vi "Stop Device.vi"(8 "error in":errorcluster, 11 "Configurable Device in":refnum<class "Configurable Device.lvclass">) -> (0 "error out":errorcluster, 3 "Configurable Device out":refnum<class "Configurable Device.lvclass">)   [LabVIEW 2014, in "Device.lvlib" / "Configurable Device.lvclass"]
uses:
  Configurable Device.lvclass
  reusable/Session APIs/File Access/Config Data/Config Data.lvclass
  reusable/Session APIs/Session Log/System Log.lvclass
  Configurable Device.lvclass/Configurable Device.ctl
  <userlib>/_Session Fwk/Session - Root.lvclass
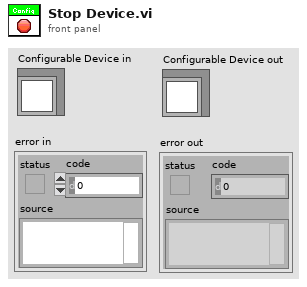
[diagram p1: front panel]
types:
  T1 = typedef "Config Data.lvclass/Config Session.ctl" = refnum<data-value>
  T2 = typedef "Session - Root.lvclass/Session Handle.ctl" = refnum<data-value>
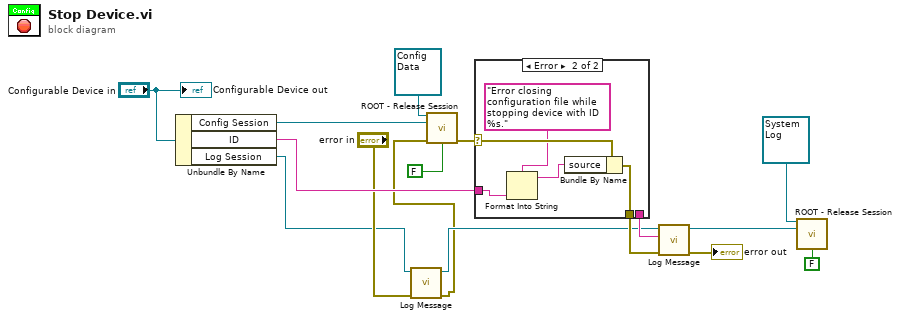
[diagram p0: block diagram]
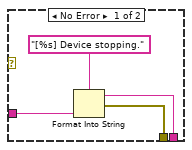
[diagram p2: hidden frame]
diagram:
  n1 = Unbundle By Name("Configurable Device in") -> ("Config Session"=w15:T1, "ID"=w13:string, "Log Session"=w3:T2)
  n2 = call "Log Message.vi"("error in"="error in", "session in"=w3) -> ("error out"=w1:errorcluster, "session out"=w2:T2)  [unwired: 8 in]
  n3 = call <userlib>:"ROOT - Release Session.vi"("OBJ - Session in"=refnum<class "Config Data.lvclass"> refnum ("Config Data"), "Session Handle in"=w15, "error in (no error)"=w1, "force destroy? (F)"=FALSE) -> ("error out"=w6:errorcluster)  [unwired: 10 in, 1 out]
  n4 = case shown="Error" w6 {
    selector: w6 -> [_ w24]
    tunnel: w13 -> [w19 w23]
    tunnel: [w18 w25] -> w12
    tunnel: [w17 _] -> w11
    frame No Error {
      n5 = Format Into String(format string="[%s] Device stopping.", w19) -> (resulting string=w17:string, error out=w18:errorcluster)  [unwired: 2 in]
    }
    frame Error {
      n6 = Format Into String(format string="Error closing configuration file while stopping device with ID %s.", w23) -> (resulting string=w21:string)  [unwired: 2 in, 1 out]
      n7 = Bundle By Name(cluster=w24, "source"=w21) -> (w25:errorcluster)
    }
  }
  n8 = call "Log Message.vi"("error in"=w12, "MSG In"=w11, "session in"=w2) -> ("error out"=→"error out":errorcluster, "session out"=w10:T2)  [unwired: 7 in]
  n9 = call <userlib>:"ROOT - Release Session.vi"("OBJ - Session in"=refnum<class "System Log.lvclass"> refnum ("Sys Log"), "Session Handle in"=w10, "force destroy? (F)"=FALSE) -> ()  [unwired: 11 in, 2 out]
  "Configurable Device out" <- "Configurable Device in"
